vi "Compute Laplacian 32f.vi"(8 "Error In":errorcluster, 10 "Input":T1 {"Dimension"."Width" min=1; "Dimension"."Height" min=1; "Dimension"."Depth" min=1}, 11 "Laplacian Object":T6 {"Laplacian Out"."Dimension"."Width" min=1; "Laplacian Out"."Dimension"."Height" min=1; "Laplacian Out"."Dimension"."Depth" min=1}) -> (0 "Error Out":errorcluster, 3 "Laplacian Out":T1 {"Dimension"."Width" min=1; "Dimension"."Height" min=1; "Dimension"."Depth" min=1}, 4 "Time in ms":dbl)   [LabVIEW 2012, in "OpenCLV x64.lvlib"]
doc: "Computes the Laplacian based on already created Laplacian Object. The dimensions of the input array <b>must</b> match the size of the dimension used to define the Laplacian Object."
uses:
  OpenCLV x64.lvlib
  Controls/Laplacian Object.ctl
  Controls/Device ID.ctl
  Controls/Program Handle.ctl
  Controls/Memory Object.ctl
  Controls/Memory ID.ctl
  User Controls/Array Dimensions.ctl
  Controls/Memory Type.ctl
  Error Checking/Add Error Functional Global.vi
  Set Kernel Arguments/Set Kernel Arguments Memory Object.vi
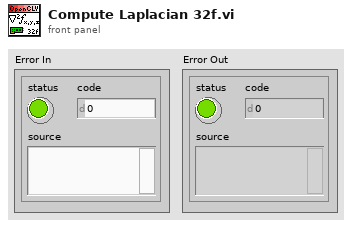
[diagram p1: front panel]
types:
  T1 = typedef "OpenCLV x64.lvlib/Memory Object.ctl" = cluster{"Device ID":T2, "Memeroy ID":T3, "Dimension":T4, "Memory Type":T5}
  T2 = typedef "OpenCLV x64.lvlib/Device ID.ctl" = u64
  T3 = typedef "OpenCLV x64.lvlib/Memory ID.ctl" = u64
  T4 = typedef "Array Dimensions.ctl" = cluster{"Depth":u64, "Height":u64, "Width":u64}
  T5 = typedef "OpenCLV x64.lvlib/Memory Type.ctl" = enum16{"32f", "u8", "i8", "u16", "i16", "u32", "i32", "64f"}
  T6 = typedef "OpenCLV x64.lvlib/Laplacian Object.ctl" = cluster{"Device Out":T2, "Program Handle":T7, "Laplacian Out":T1}
  T7 = typedef "OpenCLV x64.lvlib/Program Handle.ctl" = u64
  T8 = typedef "OpenCLV x64.lvlib/Kernel Handle.ctl" = u64
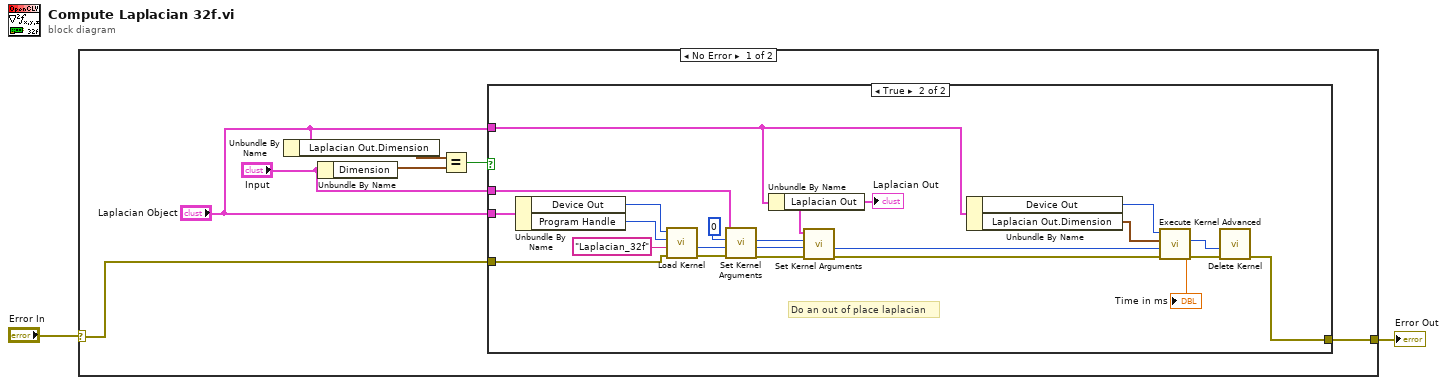
[diagram p0: block diagram]
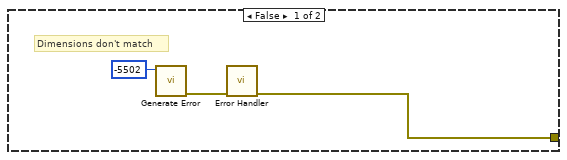
[diagram p2: hidden frame]
diagram:
  n1 = case shown="No Error" "Error In" {
    selector: "Error In" -> [w4 w35]
    tunnel: [w9 w35] -> w1
    frame No Error {
      n2 = Unbundle By Name("Laplacian Object") -> ("Laplacian Out.Dimension"=w8:T4)
      n3 = Unbundle By Name("Input") -> ("Dimension"=w7:T4)
      n4 = Equal?(x=w8, y=w7) -> (x = y?=w6:bool)
      n5 = case shown="True" w6 {
        tunnel: [w10 w34] -> w9
        tunnel: "Laplacian Object" -> [_ w15]
        tunnel: "Input" -> [_ w17]
        tunnel: w4 -> [_ w18]
        tunnel: "Laplacian Object" -> [_ w16]
        frame False {
          # "Dimensions don't match"
          n6 = call "Generate Error.vi"("Error"=-5502) -> ("error out"=w11:errorcluster)  [unwired: 10 in]
          n7 = call-poly "Error Handler.vi"("Error In"=w11) -> ("Error Out"=w10:errorcluster)  [unwired: 10 in]
        }
        frame True {
          # "Do an out of place laplacian"
          n8 = Unbundle By Name(w16) -> ("Device Out"=w22:T2, "Program Handle"=w21:T7)
          n9 = call "Load Kernel.vi"("Error In"=w18, "Kernel Name"="Laplacian_32f", "Program Handle"=w21, "Device In"=w22) -> ("Error Out"=w20:errorcluster, "Kernel Handle"=w19:T8)  [unwired: 4 in, 2 out]
          n10 = call-poly "Set Kernel Arguments.vi"("Error In"=w20, "Kernel Handle"=w19, "Argument Number"=0, "Memory Object"=w17) -> ("Error Out"=w30:errorcluster, "Kernel Handle out"=w31:T8, "Auto Inc Arugment Number"=w32:i32)  [unwired: 5 in]
          n11 = Unbundle By Name(w15) -> ("Laplacian Out"=w14:T1)
          "Laplacian Out" <- w14
          n12 = call-poly "Set Kernel Arguments.vi"("Error In"=w30, "Kernel Handle"=w31, "Argument Number"=w32, "Memory Object"=w14) -> ("Error Out"=w24:errorcluster, "Kernel Handle out"=w25:T8)  [unwired: 5 in, 1 out]
          n13 = Unbundle By Name(w15) -> ("Device Out"=w29:T2, "Laplacian Out.Dimension"=w13:T4)
          n14 = call "Execute Kernel Advanced.vi"("Error In"=w24, "Kernel Handle"=w25, "Thread Dimensions"=w13, "Device In"=w29) -> ("Error Out"=w27:errorcluster, "Kernel Handle out"=w26:T8, "Time in ms"=→"Time in ms":dbl)  [unwired: 4 in, 1 out]
          n15 = call "Delete Kernel.vi"("Error In"=w27, "Kernel In"=w26) -> ("Error Out"=w34:errorcluster)  [unwired: 9 in]
        }
      }
    }
    frame Error {
    }
  }
  "Error Out" <- w1
